vi "CPU_MEM_char_ROM.vi"(5 "init size":u16=4095, 7 "oper":enum16{"init", "read", "write"}(ring), 10 "value in":u8 format="%02x", 11 "address":u16 format="%04x") -> (2 "value out":u8 format="%02x")   [LabVIEW 2018]
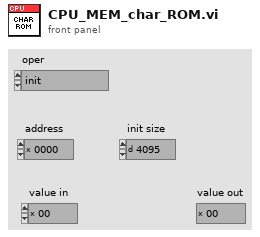
[diagram p1: front panel]
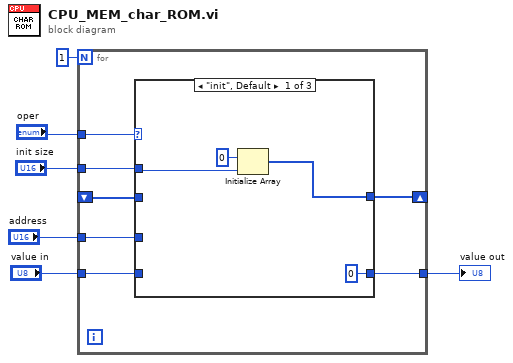
[diagram p0: block diagram]
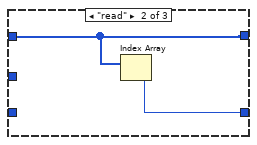
[diagram p2: hidden frame]
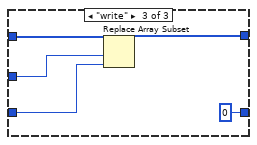
[diagram p3: hidden frame]
diagram:
  n1 = for {
    N: 1 -> [_]
    shift-right: [w11] -> _
    shift-left: _ -> [w10]
    tunnel: "oper" -> [w13]
    tunnel: "init size" -> [w12]
    tunnel: [w9] -> w3
    tunnel: "address" -> [w8]
    tunnel: "value in" -> [w7]
    n2 = case shown="\"init\", Default" w13 {
      tunnel: w12 -> [w14 _ _]
      tunnel: [w16 w19 w21] -> w11
      tunnel: w10 -> [_ w19 w24]
      tunnel: [u8 0 ("element") w18 u8 0 ("element")] -> w9
      tunnel: w8 -> [_ _ w23]
      tunnel: w7 -> [_ _ w22]
      frame "init", Default {
        n3 = Initialize Array(u8 0 ("element"), w14) -> (w16:u8[])
      }
      frame "read" {
        n4 = Index Array(array=w19) -> (element=w18:u8)  [unwired: 1 in]
      }
      frame "write" {
        n5 = Replace Array Subset(array=w24, new element=w22, index=w23) -> (w21:u8[])
      }
    }
  }
  "value out" <- w3
